vi "PH_Synchrolock_Watch.PC Set Waveform End.vi"(0 "i ref in":refnum<vi>, 2 "Waveform End":i32=10000, 5 "error in (no error)":errorcluster) -> (14 "i ref out":refnum<vi>, 19 "error out":errorcluster)   [LabVIEW 2014, in "PH_Synchrolock_Watch.lvlib"]
doc: "This is the Proc Case \"Remote Control\"."
uses:
  PH_Synchrolock_Watch.lvlib
  PH_Basics/PH_Common/PH_Common.lvlib
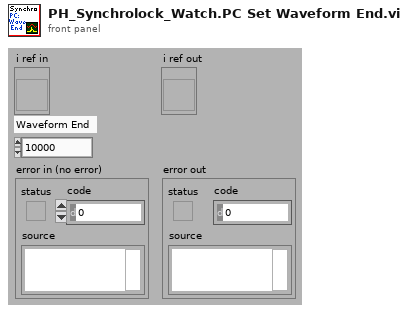
[diagram p1: front panel]
types:
  T1 = typedef "PH_Synchrolock_Watch.lvlib/PH_Synchrolock_Watch.i attribute.ctl" = cluster{"GUI Refs":cluster{"Mean Phase Graph":refnum<vi>, "RF Amplitude Graph":refnum<vi>, "Mira Amplitude Graph":refnum<vi>, "MIRA State":refnum<vi>, "Mean Phase":refnum<vi>, "RF Amplitude":refnum<vi>, "Mira Amplitude":refnum<vi>, "Mean Phase in range?":refnum<vi>, "RF Amplitude above limit?":refnum<vi>, "Mira Amplitude in range?":refnum<vi>, "Mean phase upper limit":refnum<vi>, "Mean phase lower limit":refnum<vi>, "RF Amplitude lower limit":refnum<vi>, "Mira Amplitude lower limit":refnum<vi>, "Mira Amplitude upper limit":refnum<vi>, "Waveform End":refnum<vi>, "Mira scope":refnum<vi>, "Reset Mira warning":refnum<vi>}, "Status":cluster{"Reset Warning":bool}, "Mean Phase":cluster{"Current Value":dbl, "Upper Limit":dbl, "Lower Limit":dbl, "Data":cluster{dbl[], dbl[]}}, "RF":cluster{"Current Value":dbl, "Lower Limit":dbl, "Data":cluster{dbl[], dbl[]}}, "MIRA":cluster{"Current Value":dbl, "Upper Limit":dbl, "Lower Limit":dbl, "Data":cluster{dbl[], dbl[]}}, "Waveform End":i32}
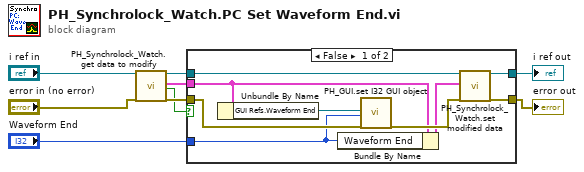
[diagram p0: block diagram]
diagram:
  n1 = call "PH_Synchrolock_Watch.get data to modify.vi"("i ref in"="i ref in", "error in (no error)"="error in (no error)") -> ("i ref out"=w9:refnum<vi>, "i attribute"=w3:T1, "timed out"=w1:bool, "error out"=w5:errorcluster)  [unwired: 14 in]
  n2 = case shown="False" w1 {
    tunnel: w9 -> [w18 w20]
    tunnel: [w17 w20] -> w6
    tunnel: w5 -> [w16 w19]
    tunnel: [w14 w19] -> w4
    tunnel: w3 -> [w12 _]
    tunnel: "Waveform End" -> [w11 _]
    frame False {
      n3 = Unbundle By Name(w12) -> ("GUI Refs.Waveform End"=w13:refnum<vi>)
      n4 = Bundle By Name(cluster=w12, "Waveform End"=w11) -> (w10:T1)
      n5 = call "PH_GUI.set I32 GUI object.vi"("I32 GUI Ref"=w13, "value"=w11, "error in (no error)"=w16) -> ("error out"=w15:errorcluster)  [unwired: 16 in]
      n6 = call "PH_Synchrolock_Watch.set modified data.vi"("i ref in"=w18, "i attribute"=w10, "error in (no error)"=w15) -> ("i ref out"=w17:refnum<vi>, "error out"=w14:errorcluster)  [unwired: 15 in]
    }
    frame True {
    }
  }
  "i ref out" <- w6
  "error out" <- w4
